vi "TextFit_Size Character array to fit.vi"(8 "Error":errorcluster, 9 "Size To Fit":i32, 11 "Character Array":T1[](array[typedef])) -> (0 "Error Out":errorcluster, 2 "Pixel Width Out":i32, 3 "Character Array Out":T1[](array[typedef]))   [LabVIEW 2014]
uses:
  Controls/Cluster/Cluster_Character Size and Priority Data.ctl
  Controls/String_Picture/String Char Normal.ctl
  Controls/Enum/ENUM_Font Size Select.ctl
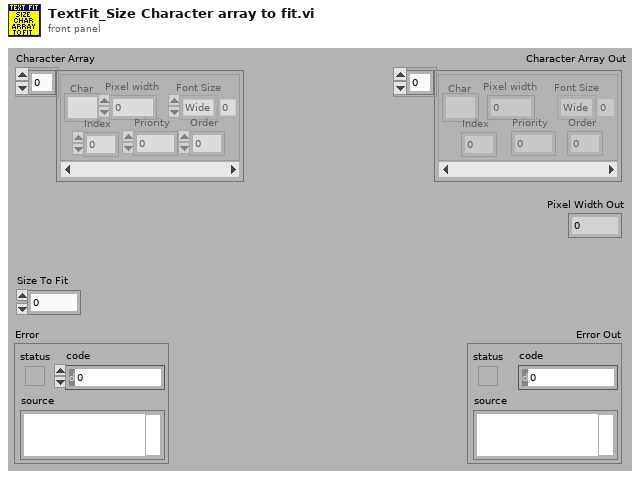
[diagram p1: front panel]
types:
  T1 = typedef "Cluster_Character Size and Priority Data.ctl" = cluster{"Char":T2, "Font Size":T3, "Pixel width":i32, "Priority":i32, "Order":i32, "Index":i32}
  T2 = typedef "String Char Normal.ctl" = string
  T3 = typedef "ENUM_Font Size Select.ctl" = enum16{"Wide", "Med", "Thin"}
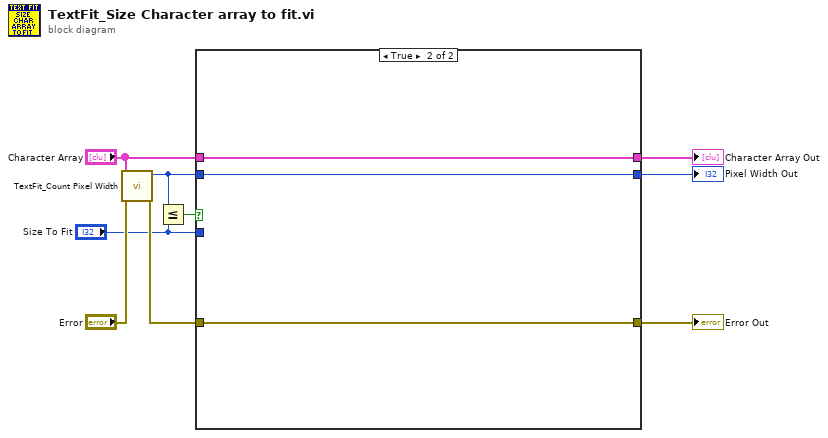
[diagram p0: block diagram]
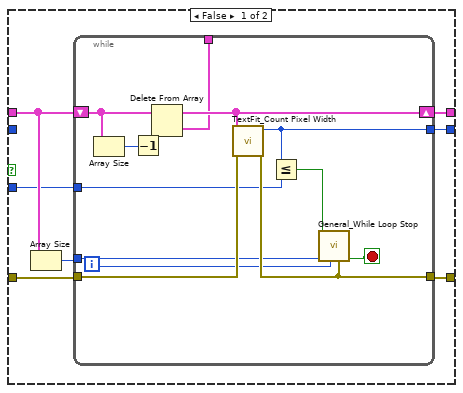
[diagram p2: hidden frame]
diagram:
  n1 = call "TextFit_Count Pixel Width.vi"("Error"="Error", "Counter Array"="Character Array") -> ("Error Out"=w5:errorcluster, "Pixel Width Out"=w1:i32)  [unwired: 8 in]
  n2 = Less Or Equal?(x=w1, y="Size To Fit") -> (x <= y?=w4:bool)
  n3 = case shown="True" w4 {
    tunnel: [w16 w31] -> w9
    tunnel: [w14 w32] -> w8
    tunnel: "Character Array" -> [w13 w32]
    tunnel: w5 -> [w12 w31]
    tunnel: "Size To Fit" -> [w11 _]
    tunnel: [w10 w30] -> w2
    tunnel: w1 -> [_ w30]
    frame False {
      n4 = Array Size(array=w13) -> (size(s)=w15:i32)
      n5 = while {
        tunnel: w12 -> [w29]
        tunnel: [w28] -> w16
        tunnel: w15 -> [w25]
        shift-right: [w24] -> w14
        shift-left: w13 -> [w23]
        tunnel: w11 -> [w20]
        tunnel: [w18] -> w10
        tunnel: [w17] -> _
        i -> [w26]
        stop <- w27 stop-if-true
        n6 = Array Size(array=w23) -> (size(s)=w22:i32)
        n7 = Decrement(x=w22) -> (x-1=w21:i32)
        n8 = Delete From Array(array=w23, index=w21) -> (deleted portion=w17:T1, array with subset deleted=w24:T1[])  [unwired: 1 in]
        n9 = call "TextFit_Count Pixel Width.vi"("Error"=w29, "Counter Array"=w24) -> ("Error Out"=w28:errorcluster, "Pixel Width Out"=w18:i32)  [unwired: 8 in]
        n10 = Less Or Equal?(x=w18, y=w20) -> (x <= y?=w19:bool)
        n11 = call "General_While Loop Stop.vi"("Error In"=w28, "Index In"=w26, "Array Size In"=w25, "Stop 1 In"=w19) -> ("Stop Out3"=w27:bool)  [unwired: 3 in, 3 out]
      }
    }
    frame True {
    }
  }
  "Error Out" <- w9
  "Pixel Width Out" <- w2
  "Character Array Out" <- w8
